vi "Icon_Size Text.vi"(7 "Rows":u32, 8 "Error":errorcluster, 11 "Text":T1[](array[typedef])) -> (0 "Error Out":errorcluster, 3 "Text Out":T1[](array[typedef]))   [LabVIEW 2009]
uses:
  Controls/String_Picture/STRING_Line Display.ctl
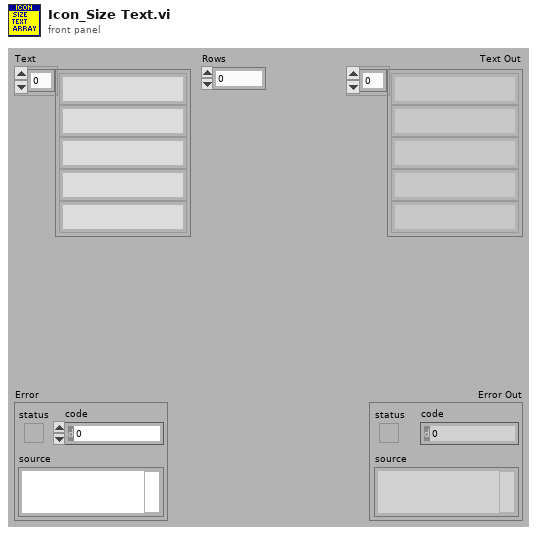
[diagram p1: front panel]
types:
  T1 = typedef "STRING_Line Display.ctl" = string
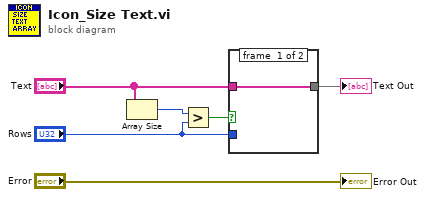
[diagram p0: block diagram]
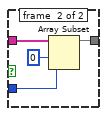
[diagram p2: hidden frame]
diagram:
  n1 = Array Size(array="Text") -> (size(s)=w6:i32)
  n2 = Greater?(x=w6, y="Rows") -> (0:w3:bool)
  n3 = case shown="True" w3 {
    tunnel: "Text" -> [w7 w11]
    tunnel: [w7 w10] -> w5
    tunnel: "Rows" -> [_ w9]
    frame #0 {
    }
    frame #1 {
      n4 = Array Subset(array=w11, index=0, length=w9) -> (w10:T1[])
    }
  }
  "Text Out" <- w5
  "Error Out" <- "Error"
